vi "Read TCPComEvents.vi"(8 "error in (no error)":errorcluster, 11 "TCPCommunicator in":refnum<class "TCPCommunicator.lvclass">) -> (0 "error out":errorcluster, 2 "TCPComEvents.lvclass":refnum<class "TCPComEvents.lvclass">, 3 "TCPCommunicator out":refnum<class "TCPCommunicator.lvclass">)   [LabVIEW 2016, in "TCPCommunicator.lvclass"]
uses:
  TCPCommunicator.lvclass
  TCPComEvents/TCPComEvents.lvclass
  TCPCommunicator.lvclass/TCPCommunicator.ctl
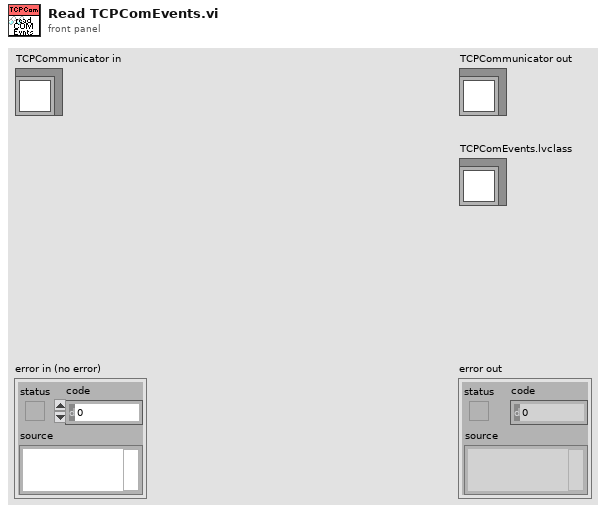
[diagram p1: front panel]
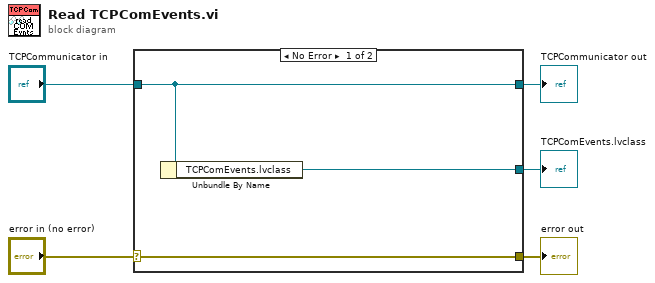
[diagram p0: block diagram]
diagram:
  n1 = case shown="No Error" "error in (no error)" {
    selector: "error in (no error)" -> [w8 w9]
    tunnel: [w8 w9] -> w4
    tunnel: [w7 w10] -> w2
    tunnel: "TCPCommunicator in" -> [w7 w10]
    tunnel: [w6 _] -> w1
    frame No Error {
      n2 = Unbundle By Name(w7) -> ("TCPComEvents.lvclass"=w6:refnum<class "TCPComEvents.lvclass">)
    }
    frame Error {
    }
  }
  "error out" <- w4
  "TCPCommunicator out" <- w2
  "TCPComEvents.lvclass" <- w1
